vi "white_key_length.get.vi"(8 "error in (no error)":errorcluster, 11 "midi-ui in":refnum<class "midi-ui.lvclass">) -> (0 "error out":errorcluster, 2 "White Key Length":dbl, 3 "midi-ui out":refnum<class "midi-ui.lvclass">)   [LabVIEW 2020, in "midi-ui.lvclass"]
uses:
  midi-ui.lvclass
  midi-ui.lvclass/midi-ui.ctl
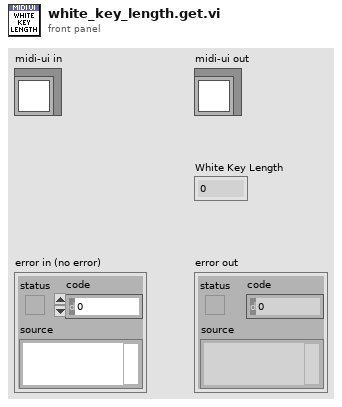
[diagram p1: front panel]
types:
  T1 = typedef "midi-ui.lvclass/privatedata.ctl" = cluster{"White Key Length":dbl, "White Key Width":dbl, "Black Key Length":dbl, "Polygon Corners by Name":map{string, cluster{"x":dbl, "y":dbl}[]}, "Anticlockwise rotations [0-3] (0)":i32, "Polygon Corners by Note Name":map{string, cluster{"x":dbl, "y":dbl}[]}, "Picture Control":refnum<vi>, "Owning VI":refnum<vi>, "Control Index":i32, "Note Bounds by Note Name":map{string, cluster{"max":dbl, "min":dbl}}, "Notes on screen":cluster{"Note Value":enum8{"C-2", "C#-2", "D-2", "D#-2", "E-2", "F-2", "F#-2", "G-2", "G#-2", "A-2", "A#-2", "B-2", "C-1", "C#-1", "D-1", "D#-1", "E-1", "F-1", "F#-1", "G-1", "G#-1", "A-1", "A#-1", "B-1", "C0", "C#0", "D0", "D#0", "E0", "F0", "F#0", "G0", "G#0", "A0", "A#0", "B0", "C1", "C#1", "D1", "D#1", "E1", "F1", "F#1", "G1", "G#1", "A1", "A#1", "B1", "C2", "C#2", "D2", "D#2", "E2", "F2", "F#2", "G2", "G#2", "A2", "A#2", "B2", "C3", "C#3", "D3", "D#3", "E3", "F3", "F#3", "G3", "G#3", "A3", "A#3", "B3", "C4", "C#4", "D4", "D#4", "E4", "F4", "F#4", "G4", "G#4", "A4", "A#4", "B4", "C5", "C#5", "D5", "D#5", "E5", "F5", "F#5", "G5", "G#5", "A5", "A#5", "B5", "C6", "C#6", "D6", "D#6", "E6", "F6", "F#6", "G6", "G#6", "A6", "A#6", "B6", "C7", "C#7", "D7", "D#7", "E7", "F7", "F#7", "G7", "G#7", "A7", "A#7", "B7", "C8", "C#8", "D8", "D#8", "E8", "F8", "F#8", "G"}, "End Time":u32, "Start Time":u32}[], "Polygon Pictures by Note Name":map{i32, cluster{"Note On":picture, "Note Off":picture}}, "keyboard":picture[], "Keyboard Note Index by Name":map{i32, i32}, "music":picture[]}
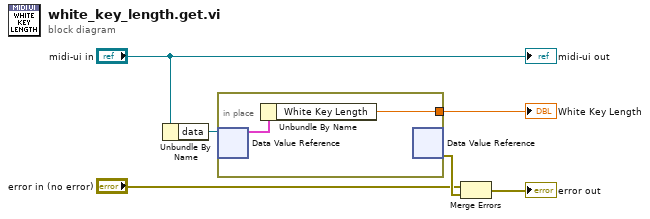
[diagram p0: block diagram]
diagram:
  n1 = Unbundle By Name("midi-ui in") -> ("data"=w6:refnum<data-value>)
  n2 = in-place {
    in-place-border: [w7] -> w1
    n3 = in-place-dvr #1(w6) -> (w8:T1)  [unwired: 1 out]
    n4 = Unbundle By Name(w8) -> ("White Key Length"=w7:dbl)
    n5 = in-place-dvr #1() -> (w4:errorcluster)  [unwired: 1 in, 1 out]
  }
  "White Key Length" <- w1
  n6 = Merge Errors("error in (no error)", w4) -> (→"error out":errorcluster)
  "midi-ui out" <- "midi-ui in"
